vi "GenerateReceipt.vi"(8 "error in (no error)":errorcluster, 11 "STOMP in":refnum<class "STOMP.lvclass">) -> (0 "error out":errorcluster, 2 "Receipt Header":T1, 3 "STOMP out":refnum<class "STOMP.lvclass">)   [LabVIEW 2017, in "STOMP.lvclass"]
uses:
  STOMP.lvclass
  Typedefs/Type_FrameHeader.ctl
  STOMP.lvclass/STOMP.ctl
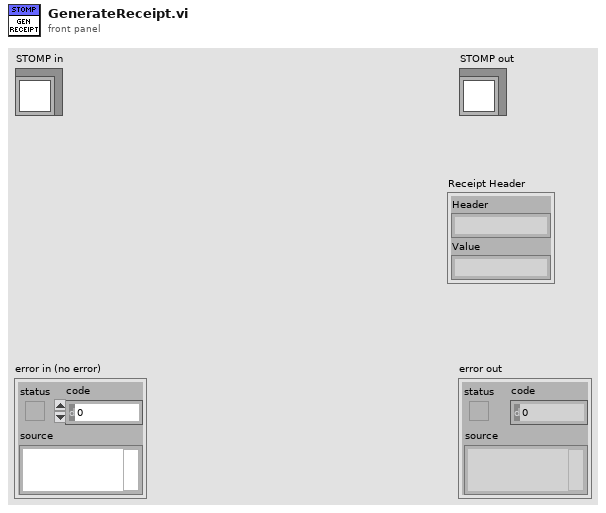
[diagram p1: front panel]
types:
  T1 = typedef "STOMP.lvclass/Type_FrameHeader.ctl" = cluster{"Header":string, "Value":string}
  T2 = typedef "LabVIEW STOMP.lvlib/STOMP.lvclass/ObjectAttributes.ctl" = cluster{"address":string, "port":u16, "ConnectionRef":refnum<k5>, "messageQueue":refnum<queue>, "receiptQueue":refnum<queue>, "errorQueue":refnum<queue>, "sendQueue":refnum<queue>, "currentReceiptNumber":u64, "currentSubscriptionId":u64, "closeConnection":bool, "activeSubscriptions":T3[]}
  T3 = typedef "Type_ActiveSubscription.ctl" = cluster{"id":u64, "receipt":bool, "Destination":string, "ack":T4, "headers":T5[]}
  T4 = typedef "Type_AckHeader.ctl" = enum16{"auto", "client", "client-individual"}
  T5 = typedef "LabVIEW STOMP.lvlib/STOMP.lvclass/Type_FrameHeader.ctl" = cluster{"Header":string, "Value":string}
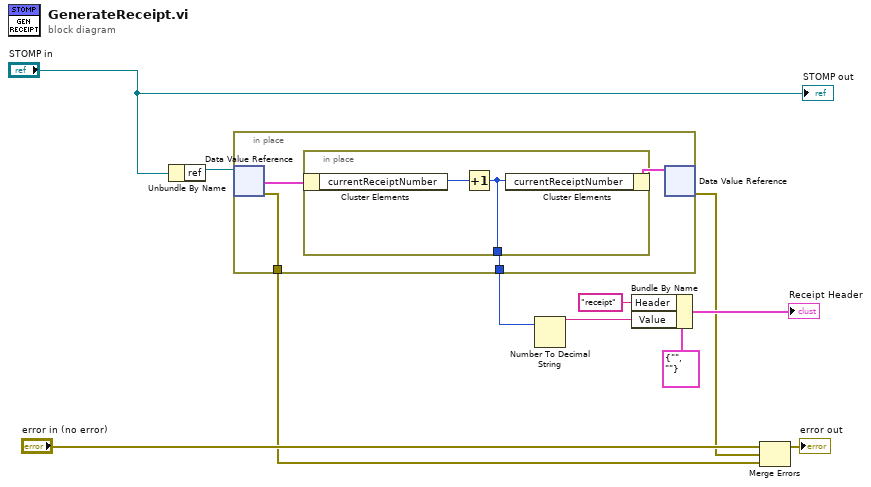
[diagram p0: block diagram]
diagram:
  n1 = Unbundle By Name("STOMP in") -> ("ref"=w5:refnum<data-value>)
  n2 = in-place {
    in-place-border: [w15] -> w7
    in-place-border: [w12] -> w1
    n3 = in-place-dvr #1(w5) -> (w14:T2, w12:errorcluster)
    n4 = in-place {
      in-place-border: [w16] -> w15
      n5 = in-place-cluster #2(w14) -> ("currentReceiptNumber"=w17:u64)
      n6 = Increment(x=w17) -> (x+1=w16:u64)
      n7 = in-place-cluster #2("currentReceiptNumber"=w16) -> (w13:T2)
    }
    n8 = in-place-dvr #1(w13) -> (w2:errorcluster)  [unwired: 1 out]
  }
  n9 = Number To Decimal String(number=w7) -> (decimal integer string=w6:string)  [unwired: 1 in]
  n10 = Bundle By Name(cluster=T1 {"Header"="", "Value"=""} ("Type_FrameHeader"), "Header"="receipt", "Value"=w6) -> (→"Receipt Header":T1)
  n11 = Merge Errors("error in (no error)", w2, w1) -> (→"error out":errorcluster)
  "STOMP out" <- "STOMP in"
